vi "Material-ChoosePart#-Spec.vi"(8 "error in (no error)":errorcluster, 11 "Material-RunTest.lvclass":refnum<class "Material-RunTest.lvclass">) -> (0 "error out":errorcluster, 1 "Cancel Test":bool, 2 "Invalid Spec Values":bool, 3 "Material-RunTest.lvclass out":refnum<class "Material-RunTest.lvclass">)   [LabVIEW 2014, in "Material-RunTest.lvclass"]
uses:
  Material-RunTest.lvclass
  Material-RunTest.lvclass/Material-RunTest.ctl
  <vilib>/addons/database/Connection.llb/DB Tools Open Connec (Path).vi
  <userlib>/_OpenG.lib/array/array.llb/Search 1D Array (String)__ogtk.vi
  <userlib>/_OpenG.lib/array/array.llb/Delete Elements from 1D Array (String)__ogtk.vi
  <vilib>/Utility/error.llb/Error Cluster From Error Code.vi
  <vilib>/ErrorRing/Error Ring.xnode
  <vilib>/addons/database/NI_Database_API.lvlib
panel:
  in  "Test Operator":string
  in  "Lot Number":string
  in  "Cancel Test":bool
  in  "Choose Part":bool
  out "ZMaximum Thickness":dbl format="%_5g"
  out "ZMinimum Thickness":dbl format="%_5g"
  out "ZNominal Thickness":dbl format="%_5g"
  in  "Part Number to Search For":string
  in  "Cancel Search":bool
  in  "Search Button":bool
  in  "Part Numbers":i32(listbox)
  # "Please Enter Required Info Below"
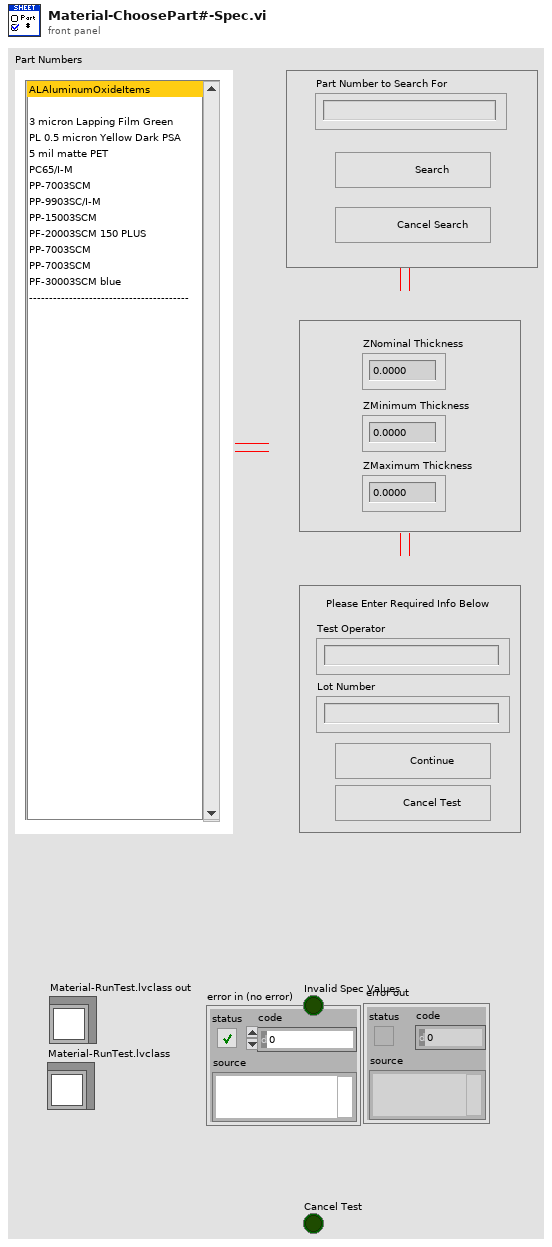
[diagram p1: front panel]
types:
  T1 = typedef "NI_Database_API.lvlib/Conn ObjectReference.ctl" = refnum<k1>
  T2 = enum8{"Enabled", "Disabled", "Disabled and Grayed Out"}
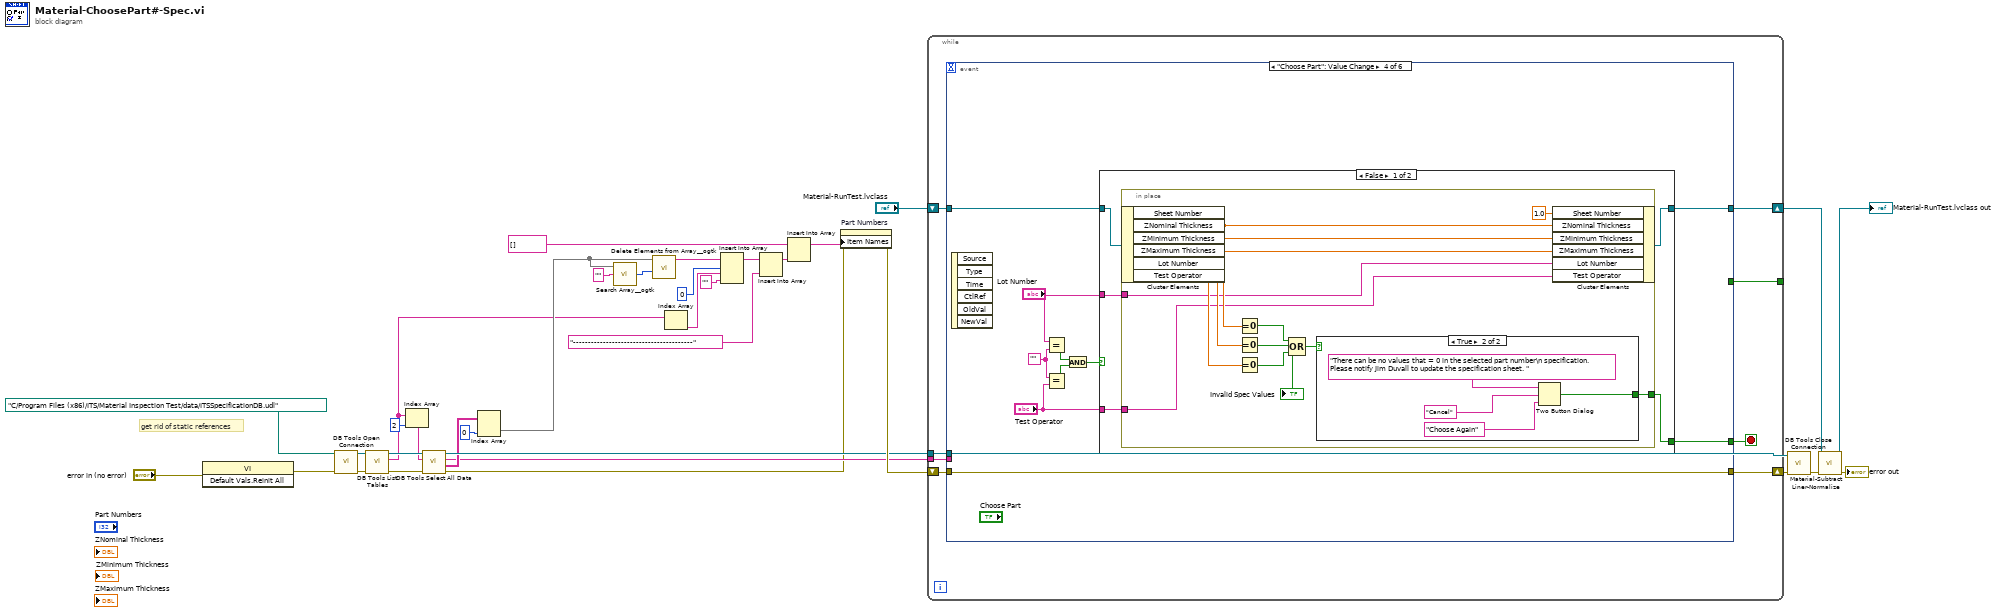
[diagram p0: block diagram]
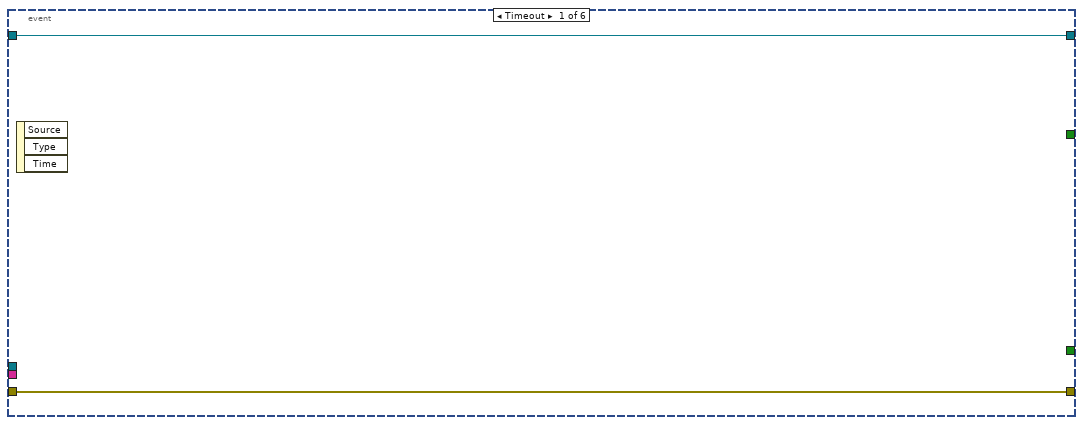
[diagram p2: hidden frame]
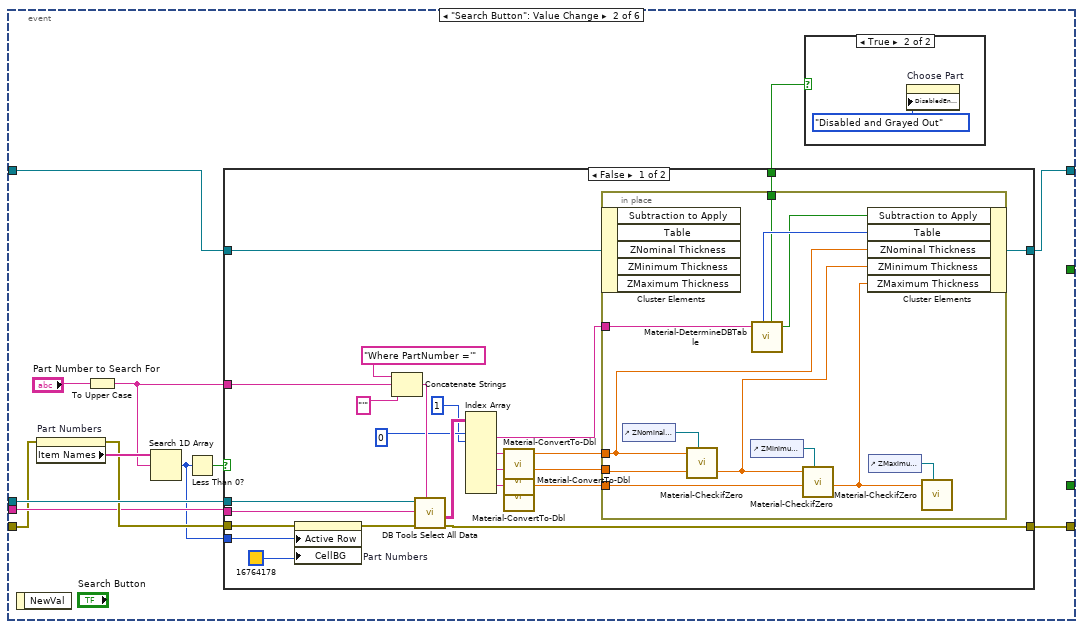
[diagram p3: hidden frame]
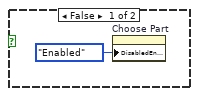
[diagram p4: hidden frame]
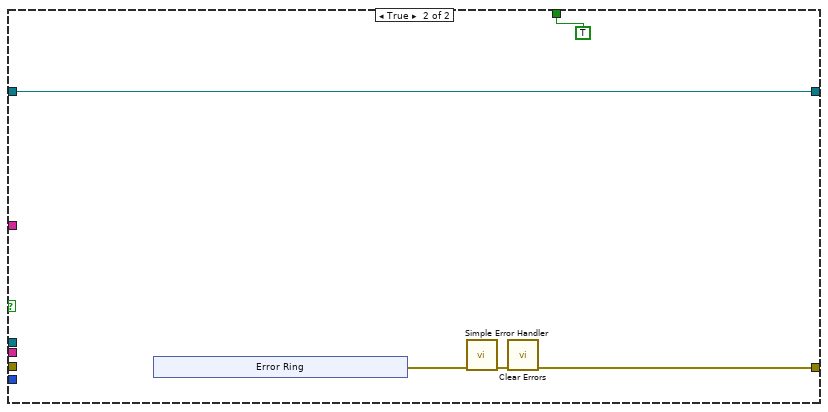
[diagram p5: hidden frame]
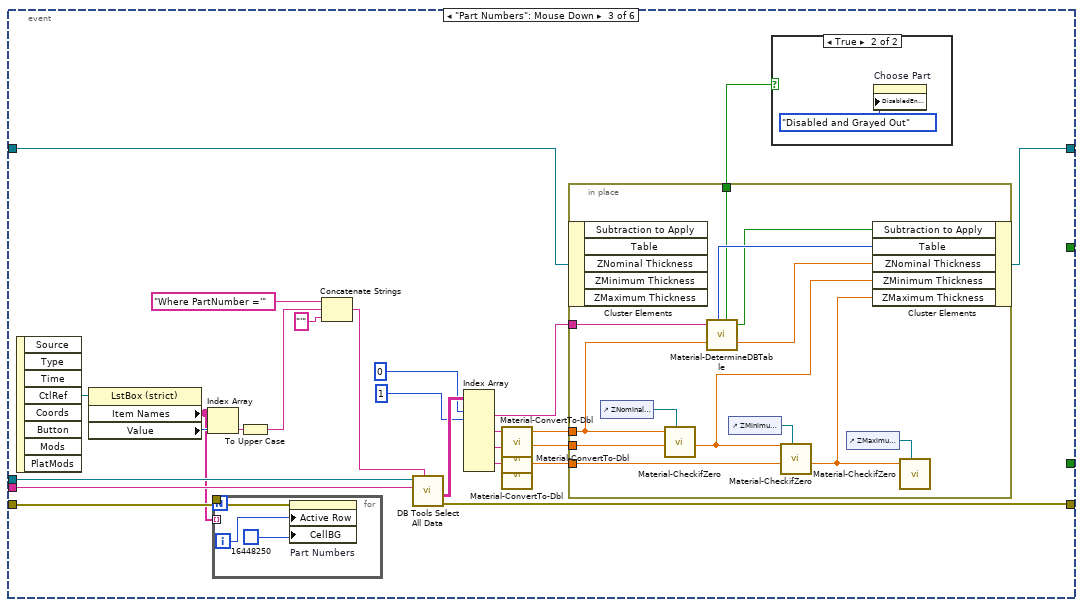
[diagram p6: hidden frame]
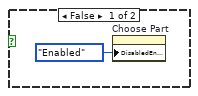
[diagram p7: hidden frame]
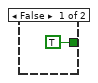
[diagram p8: hidden frame]
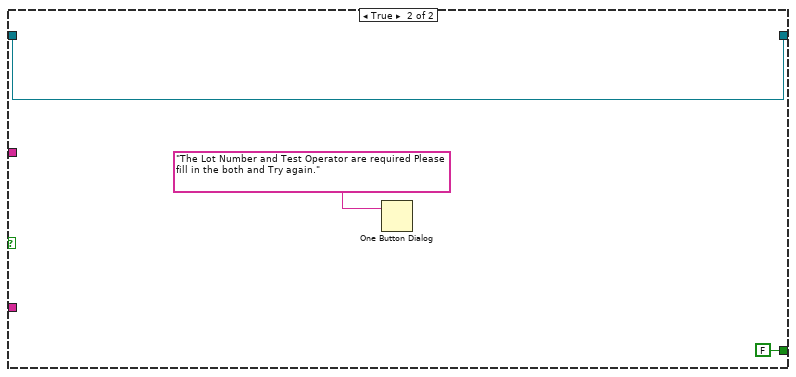
[diagram p9: hidden frame]
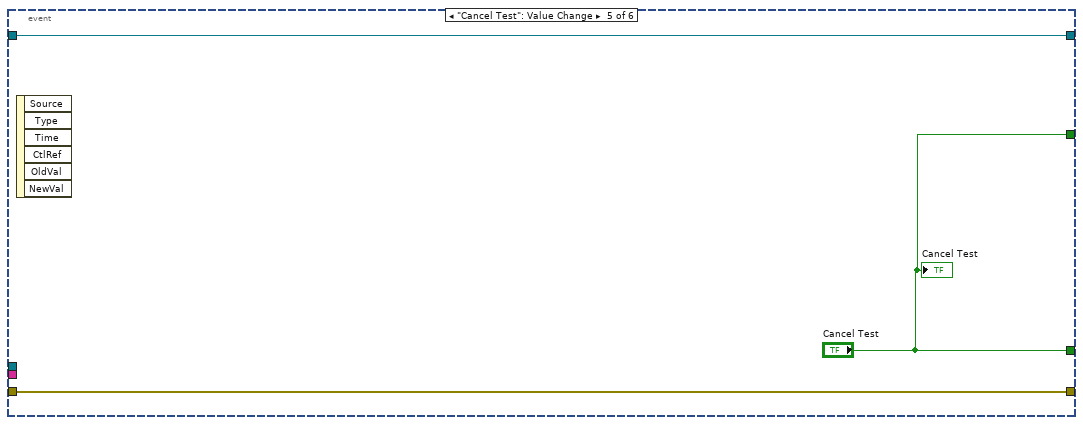
[diagram p10: hidden frame]
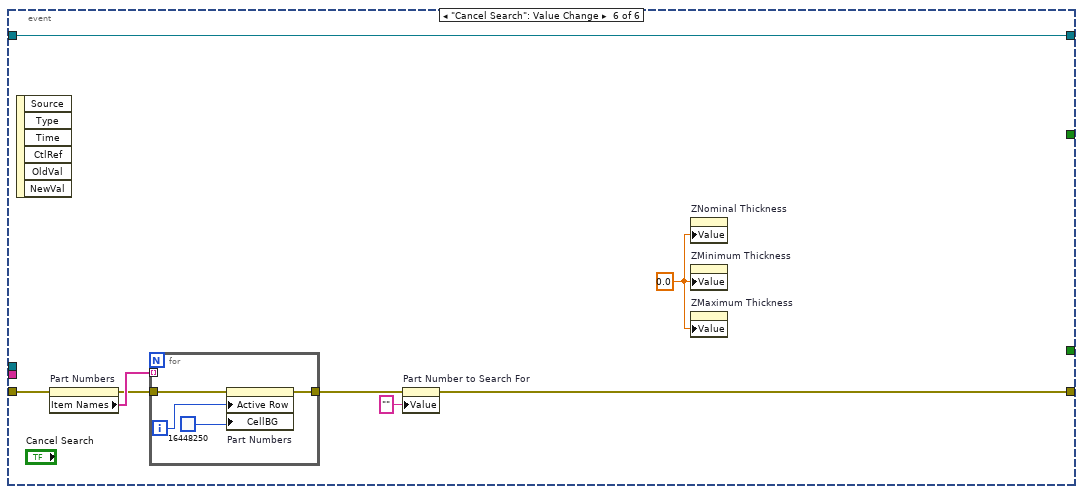
[diagram p11: hidden frame]
diagram:
  # "get rid of static references"
  n1 = invoke class="VI" method="Default Vals.Reinit All"(error in="error in (no error)") -> (error out=w24:errorcluster)  [unwired: 2 in, 2 out]
  n2 = call-poly <vilib>:"DB Tools Open Connection.vi"("error in (no error)"=w24, "connection information"=path "C:/Program Files (x86)/ITS/Material Inspection Test/data/ITSSpecificationDB.udl") -> ("error out"=w32:errorcluster, "connection reference"=w31:T1)  [unwired: 6 in]
  n3 = call <vilib>:"DB Tools List Tables.vi"("error in (no error)"=w32, "connection reference"=w31) -> ("error out"=w29:errorcluster, "tables"=w13:string[], "connection reference out"=w30:T1)  [unwired: 3 in]
  n4 = Index Array(array=w13, index=2) -> (element=w11:string)
  n5 = call <vilib>:"DB Tools Select All Data.vi"("error in (no error)"=w29, "table"=w11, "connection reference"=w30) -> ("error out"=w1:errorcluster, "data"=w15:string[][], "connection reference out"=w23:T1)  [unwired: 3 in]
  n6 = Index Array(array=w15, index (col)=0 ("disabled index (col)")) -> (element=w27:string[])  [unwired: 1 in]
  n7 = call-poly <userlib>:"Search Array__ogtk.vi"("Array"=w27, "Element Data"="") -> ("Indices of Elements"=w7:i32[])  [unwired: 7 in]
  n8 = call-poly <userlib>:"Delete Elements from Array__ogtk.vi"("indices"=w7, "array"=w27) -> ("array w/ subset deleted"=w6:string[])  [unwired: 8 in, 1 out]
  n9 = Index Array(array=w13) -> (element=w4:string)  [unwired: 1 in]
  n10 = Insert Into Array(array=w6, index=0, new element #1=w4, new element #2="" ("new element/subarray")) -> (w3:string[])
  n11 = Insert Into Array(array=w3, new element="----------------------------------------" ("new element/subarray")) -> (w9:string[])  [unwired: 1 in]
  n12 = Insert Into Array(array=string[] [], new element=w9) -> (w26:string[])  [unwired: 1 in]
  n13 = property on="Part Numbers" class="LstBox (strict)"(error in=w1, "Item Names"=w26) -> (error out=w25:errorcluster)  [unwired: 1 in, 1 out]
  n14 = while {
    tunnel: w23 -> [w41]
    tunnel: w11 -> [w40]
    shift-right: [w39] -> w20
    shift-left: w25 -> [w38]
    tunnel: [w34] -> _
    shift-right: [w35] -> w18
    shift-left: "Material-RunTest.lvclass" -> [w36]
    stop <- w37 stop-if-true
    n15 = event shown="[3] \"Choose Part\": Value Change" {
      selector: _ -> [_ _ _ _ _ _]
      dyn-events: _ -> [_ _ _ _ _ _]
      timeout: _ -> [_ _ _ _ _ _]
      tunnel: w41 -> [_ w53 w120 _ _ _]
      tunnel: w40 -> [_ w51 w119 _ _ _]
      tunnel: [w43 w50 w118 w152 w179 w187] -> w39
      tunnel: w38 -> [w43 w48 w106 w152 w179 w182]
      tunnel: [_ _ _ w151 "Cancel Test" _] -> w37
      tunnel: w36 -> [w42 w47 w117 w150 w178 w185]
      tunnel: [w42 w46 w116 w149 w178 w185] -> w35
      tunnel: [_ _ _ _ "Cancel Test" _] -> w34
      event Timeout {
        n16 = event-data() -> ()  [unwired: 1 in, 3 out]
      }
      event "Search Button": Value Change {
        n17 = event-data() -> ()  [unwired: 1 in, 1 out]
        n18 = property on="Part Numbers" class="LstBox (strict)"(error in=w48) -> (error out=w52:errorcluster, "Item Names"=w56:string[])  [unwired: 1 in, 1 out]
        n19 = To Upper Case(1:"Part Number to Search For") -> (0:w49:string)
        n20 = Search 1D Array(1D array=w56, element=w49) -> (index of element=w45:i32)  [unwired: 1 in]
        n21 = Less Than 0?(x=w45) -> (x < 0?=w54:bool)
        n22 = case shown="False" w54 {
          tunnel: w53 -> [w82 _]
          tunnel: w52 -> [w64 _]
          tunnel: w51 -> [w81 _]
          tunnel: [w76 w95] -> w50
          tunnel: w49 -> [w79 _]
          tunnel: w47 -> [w75 w94]
          tunnel: [w74 w94] -> w46
          tunnel: w45 -> [w62 _]
          tunnel: [w59 TRUE ("Unique identifier isn't present")] -> w44
          frame False {
            n23 = property on="Part Numbers" class="LstBox (strict)"(error in=w64, "Active Row"=w62, "CellBG"=u32 16764178) -> (error out=w63:errorcluster)  [unwired: 1 in, 1 out]
            n24 = Concatenate Strings("Where PartNumber ='" ("optional clause"), w79, "'" ("string")) -> (w77:string)
            n25 = call <vilib>:"DB Tools Select All Data.vi"("optional clause"=w77, "error in (no error)"=w63, "table"=w81, "connection reference"=w82) -> ("error out"=w76:errorcluster, "data"=w73:string[][])  [unwired: 2 in, 1 out]
            n26 = Index Array(array=w73, index (row) #1=0 ("disabled index (row)"), index (col) #1=1 ("disabled index (col)")) -> (element #1=w60:string, element #2=w72:string, element #3=w71:string, element #4=w70:string)  [unwired: 6 in]
            n27 = call "Material-ConvertTo-Dbl.vi"("DBL String"=w72) -> ("DBL liner out"=w69:dbl)  [unwired: 8 in]
            n28 = call "Material-ConvertTo-Dbl.vi"("DBL String"=w71) -> ("DBL liner out"=w68:dbl)  [unwired: 8 in]
            n29 = call "Material-ConvertTo-Dbl.vi"("DBL String"=w70) -> ("DBL liner out"=w67:dbl)  [unwired: 8 in]
            n30 = in-place {
              in-place-border: w69 -> [w91]
              in-place-border: w68 -> [w89]
              in-place-border: w67 -> [w88]
              in-place-border: w60 -> [w86]
              in-place-border: [w84] -> w59
              n31 = in-place-cluster #1(w75) -> ()  [unwired: 5 out]
              n32 = control-ref of="ZNominal Thickness"() -> (w92:refnum<vi>)
              n33 = call "Material-CheckifZero.vi"("DBL liner in"=w91, "Digital in"=w92) -> ()  [unwired: 9 in]
              n34 = control-ref of="ZMinimum Thickness"() -> (w90:refnum<vi>)
              n35 = call "Material-DetermineDBTable.vi"("Description"=w86) -> ("Table Number Out"=w85:i32, "Unique identifier isn't present"=w84:bool, "Subtraction to Choose"=w83:bool)  [unwired: 6 in]
              n36 = call "Material-CheckifZero.vi"("DBL liner in"=w89, "Digital in"=w90) -> ()  [unwired: 9 in]
              n37 = in-place-cluster #1("Subtraction to Apply"=w83, "Table"=w85, "ZNominal Thickness"=w91, "ZMinimum Thickness"=w89, "ZMaximum Thickness"=w88) -> (w74:refnum<class "Material-RunTest.lvclass">)
              n38 = control-ref of="ZMaximum Thickness"() -> (w87:refnum<vi>)
              n39 = call "Material-CheckifZero.vi"("DBL liner in"=w88, "Digital in"=w87) -> ()  [unwired: 9 in]
            }
          }
          frame True {
            n40 = xnode "Error Ring"() -> ("error out"=w97:errorcluster)
            n41 = call <vilib>:"Simple Error Handler.vi"("error in (no error)"=w97) -> ("error out"=w96:errorcluster)  [unwired: 4 in, 4 out]
            n42 = call <vilib>:"Clear Errors.vi"("error in (no error)"=w96) -> ("error out"=w95:errorcluster)  [unwired: 5 in, 1 out]
          }
        }
        n43 = case shown="True" w44 {
          frame False {
            n44 = property on="Choose Part" class="Bool"("DisabledEnum"=T2."Enabled" ("Disabled")) -> ()  [unwired: 2 in, 2 out]
          }
          frame True {
            n45 = property on="Choose Part" class="Bool"("DisabledEnum"=T2."Disabled and Grayed Out" ("Disabled")) -> ()  [unwired: 2 in, 2 out]
          }
        }
      }
      event "Part Numbers": Mouse Down {
        n46 = event-data() -> ("CtlRef"=w127:refnum<vi>)  [unwired: 1 in, 7 out]
        n47 = property class="LstBox (strict)"(reference=w127) -> ("Item Names"=w105:string[], "Value"=w126:i32)  [unwired: 1 in, 2 out]
        n48 = Index Array(array=w105, index=w126) -> (element=w122:string)
        n49 = for {
          tunnel: w106 -> [w131]
          tunnel: w105 -> [_] mode=indexing
          i -> [w130]
          n50 = property on="Part Numbers" class="LstBox (strict)"(error in=w131, "Active Row"=w130, "CellBG"=u32 16448250) -> ()  [unwired: 1 in, 2 out]
        }
        n51 = To Upper Case(1:w122) -> (0:w121:string)
        n52 = Concatenate Strings("Where PartNumber ='" ("optional clause"), w121, "'" ("string")) -> (w123:string)
        n53 = call <vilib>:"DB Tools Select All Data.vi"("optional clause"=w123, "table"=w119, "connection reference"=w120) -> ("error out"=w118:errorcluster, "data"=w109:string[][])  [unwired: 3 in, 1 out]
        n54 = Index Array(array=w109, index (row) #1=0 ("disabled index (row)"), index (col) #1=1 ("disabled index (row)")) -> (element #1=w104:string, element #2=w115:string, element #3=w114:string, element #4=w113:string)  [unwired: 6 in]
        n55 = call "Material-ConvertTo-Dbl.vi"("DBL String"=w115) -> ("DBL liner out"=w112:dbl)  [unwired: 8 in]
        n56 = call "Material-ConvertTo-Dbl.vi"("DBL String"=w114) -> ("DBL liner out"=w111:dbl)  [unwired: 8 in]
        n57 = call "Material-ConvertTo-Dbl.vi"("DBL String"=w113) -> ("DBL liner out"=w110:dbl)  [unwired: 8 in]
        n58 = in-place {
          in-place-border: w112 -> [w139]
          in-place-border: w111 -> [w138]
          in-place-border: w110 -> [w137]
          in-place-border: w104 -> [w136]
          in-place-border: [w134] -> w103
          n59 = in-place-cluster #2(w117) -> ()  [unwired: 5 out]
          n60 = control-ref of="ZNominal Thickness"() -> (w142:refnum<vi>)
          n61 = call "Material-CheckifZero.vi"("DBL liner in"=w139, "Digital in"=w142) -> ()  [unwired: 9 in]
          n62 = call "Material-DetermineDBTable.vi"("Description"=w136) -> ("Table Number Out"=w135:i32, "Unique identifier isn't present"=w134:bool, "Subtraction to Choose"=w133:bool)  [unwired: 6 in]
          n63 = control-ref of="ZMinimum Thickness"() -> (w141:refnum<vi>)
          n64 = call "Material-CheckifZero.vi"("DBL liner in"=w138, "Digital in"=w141) -> ()  [unwired: 9 in]
          n65 = control-ref of="ZMaximum Thickness"() -> (w140:refnum<vi>)
          n66 = in-place-cluster #2("Subtraction to Apply"=w133, "Table"=w135, "ZNominal Thickness"=w139, "ZMinimum Thickness"=w138, "ZMaximum Thickness"=w137) -> (w116:refnum<class "Material-RunTest.lvclass">)
          n67 = call "Material-CheckifZero.vi"("DBL liner in"=w137, "Digital in"=w140) -> ()  [unwired: 9 in]
        }
        n68 = case shown="True" w103 {
          frame False {
            n69 = property on="Choose Part" class="Bool"("DisabledEnum"=T2."Enabled" ("Disabled")) -> ()  [unwired: 2 in, 2 out]
          }
          frame True {
            n70 = property on="Choose Part" class="Bool"("DisabledEnum"=T2."Disabled and Grayed Out" ("Disabled")) -> ()  [unwired: 2 in, 2 out]
          }
        }
      }
      event "Choose Part": Value Change {
        w147 = ""
        n71 = event-data() -> ()  [unwired: 1 in, 6 out]
        n72 = Equal?(x="Lot Number", y=w147) -> (x = y?=w146:bool)
        n73 = Equal?(x=w147, y="Test Operator") -> (x = y?=w145:bool)
        n74 = And(x=w146, y=w145) -> (x .and. y?=w144:bool)
        n75 = case shown="False" w144 {
          tunnel: w150 -> [w157 w174]
          tunnel: [w156 w174] -> w149
          tunnel: [w155 FALSE ("T button?")] -> w151
          tunnel: "Lot Number" -> [w154 _]
          tunnel: "Test Operator" -> [w153 _]
          frame False {
            n76 = in-place {
              in-place-border: [w161] -> w155
              in-place-border: w154 -> [w160]
              in-place-border: w153 -> [w158]
              n77 = in-place-cluster #3(w157) -> ("ZNominal Thickness"=w168:dbl, "ZMinimum Thickness"=w167:dbl, "ZMaximum Thickness"=w166:dbl)  [unwired: 3 out]
              n78 = Equal To 0?(x=w168) -> (x = 0?=w165:bool)
              n79 = Equal To 0?(x=w167) -> (x = 0?=w164:bool)
              n80 = Equal To 0?(x=w166) -> (x = 0?=w163:bool)
              n81 = Compound Arithmetic op=OR(w165, w164, w163) -> (w162:bool)
              "Invalid Spec Values" <- w162
              n82 = case shown="True" w162 {
                tunnel: [TRUE ("T button?") w170] -> w161
                frame False {
                }
                frame True {
                  n83 = Two Button Dialog(message="There can be no values that = 0 in the selected part number\n specification. Please notify Jim Duvall to update the specification sheet. " ("T button name (\"OK\")"), 1:"Choose Again" ("T button name (\"OK\")"), 2:"Cancel" ("F button name (\"Cancel\")")) -> (T button?=w170:bool)
                }
              }
              n84 = in-place-cluster #3("Sheet Number"=1.0, "ZNominal Thickness"=w168, "ZMinimum Thickness"=w167, "ZMaximum Thickness"=w166, "Lot Number"=w160, "Test Operator"=w158) -> (w156:refnum<class "Material-RunTest.lvclass">)
            }
          }
          frame True {
            n85 = One Button Dialog(message="The Lot Number and Test Operator are required Please fill in the both and Try again.") -> ()  [unwired: 1 in, 1 out]
          }
        }
      }
      event "Cancel Test": Value Change {
        n86 = event-data() -> ()  [unwired: 1 in, 6 out]
        "Cancel Test" <- "Cancel Test"
      }
      event "Cancel Search": Value Change {
        w180 = 0.0 ("ZMinimum Thickness")
        n87 = event-data() -> ()  [unwired: 1 in, 6 out]
        n88 = property on="Part Numbers" class="LstBox (strict)"(error in=w182) -> (error out=w181:errorcluster, "Item Names"=w183:string[])  [unwired: 1 in, 1 out]
        n89 = for {
          tunnel: w181 -> [w188]
          tunnel: [w189] -> w184
          tunnel: w183 -> [_] mode=indexing
          i -> [w190]
          n90 = property on="Part Numbers" class="LstBox (strict)"(error in=w188, "Active Row"=w190, "CellBG"=u32 16448250) -> (error out=w189:errorcluster)  [unwired: 1 in, 1 out]
        }
        n91 = property on="Part Number to Search For" class="Str"(error in=w184, "Value"="" ("Part Number to Search For")) -> (error out=w187:errorcluster)  [unwired: 1 in, 1 out]
        n92 = property on="ZNominal Thickness" class="DigNum (strict)"("Value"=w180) -> ()  [unwired: 2 in, 2 out]
        n93 = property on="ZMinimum Thickness" class="DigNum (strict)"("Value"=w180) -> ()  [unwired: 2 in, 2 out]
        n94 = property on="ZMaximum Thickness" class="DigNum (strict)"("Value"=w180) -> ()  [unwired: 2 in, 2 out]
      }
    }
  }
  n95 = call <vilib>:"DB Tools Close Connection.vi"("error in (no error)"=w20, "connection reference"=w23) -> ("error out"=w19:errorcluster)  [unwired: 5 in]
  n96 = call "Material-SubtractLiner-Normalize.vi"("error in (no error)"=w19, "Material-RunTest in"=w18) -> ("error out"=→"error out":errorcluster, "Material-RunTest out"=→"Material-RunTest.lvclass out":refnum<class "Material-RunTest.lvclass">)  [unwired: 8 in]
